vi "LI-U8 - modulus ver2.vi"(3 "Large number - U8 B":T1, 5 "Large number - U8 A":T1) -> (0 "# multiples":T1, 1 "A mod (B)":T1)   [LabVIEW 2012]
doc: "Determines modulus or division remainder of two large numbers (U8 array format).\n\nIterative procedure\na - Is A bigger than B (do subtraction)\n No - output A\n Yes - find the \"base multiplier\" of (A-B) /B . This is done by rounding A-B down so it only keeps highest digit (in base 256) and rounding B up in the same fashion, and dividing the two. Then subtract B * base multiplier from A and go back to top of the loop."
uses:
  User Access Type defs/Large number - U8 array.ctl
panel:
  out "ratio of MSDs":u8
  out "Max # shifts (U8)":u8
  out "Overflow?":bool
  out "A-B":T1
  out "iteration":i32
  # "index 0 = LSD"
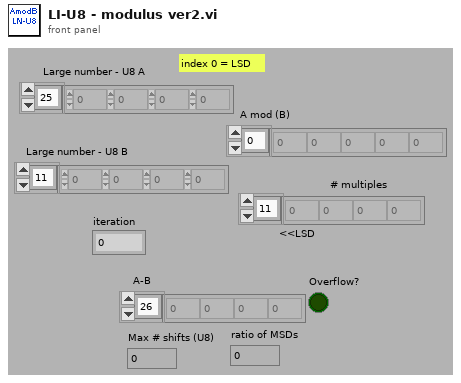
[diagram p1: front panel]
types:
  T1 = typedef "Large number - U8 array.ctl" = u8[]
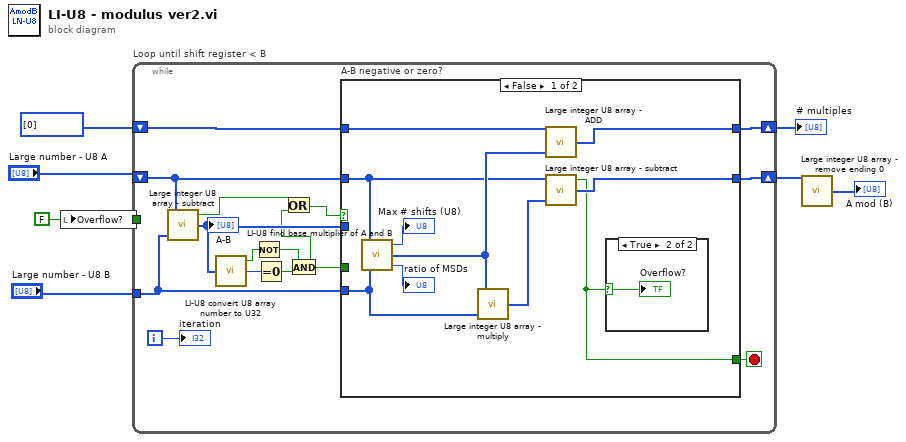
[diagram p0: block diagram]
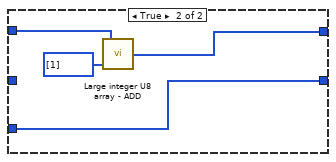
[diagram p4: hidden frame]
diagram:
  w1 = FALSE ("Overflow?")
  n1 = local write "Overflow?"(w1) -> ()
  n2 = while "Loop until shift register < B" {
    shift-right: [w22] -> w5
    shift-left: "Large number - U8 A" -> [w19]
    tunnel: "Large number - U8 B" -> [w21]
    shift-right: [w17] -> w2
    shift-left: T1 [0] ("# multiples") -> [w18]
    tunnel: w1 -> [_]
    i -> [w20]
    stop <- w8 stop-if-true
    n3 = call "Large integer U8 array - subtract.vi"("Large number - U8 B"=w21, "Large number - U8 A"=w19) -> ("A-B"=w16:T1, "Overflow?"=w11:bool)  [unwired: 2 out]
    "A-B" <- w16
    n4 = call "LI-U8 convert U8 array number to U32.vi"("Large number -U8"=w16) -> ("U32"=w15:u32, "Roll-over?"=w14:bool)  [unwired: 3 out]
    n5 = Not(x=w14) -> (.not. x?=w12:bool)
    n6 = Equal To 0?(x=w15) -> (x = 0?=w13:bool)
    n7 = And(x=w12, y=w13) -> (x .and. y?=w10:bool)
    n8 = Or(x=w11, y=w10) -> (x .or. y?=w9:bool)
    n9 = case "A-B negative or zero?" shown="False" w9 {
      selector: w9 -> [_ w34]
      tunnel: [w32 w38] -> w22
      tunnel: w19 -> [w23 w35]
      tunnel: w16 -> [_ w39]
      tunnel: w21 -> [w29 _]
      tunnel: [w30 w36] -> w17
      tunnel: w18 -> [w31 w37]
      tunnel: w10 -> [_ w40]
      tunnel: [w27 w34] -> w8
      frame False {
        n10 = call "LI-U8 find base multiplier of A and B.vi"("Large number - U8 B"=w29, "Large number - U8 A"=w23) -> ("ratio of MSDs"=→"ratio of MSDs":u8, "base multiplier"=w28:T1, "Max # shifts (U8)"=→"Max # shifts (U8)":u8)  [unwired: 1 out]
        n11 = call "Large integer U8 array - multiply.vi"("Large number - U8 2"=w29, "Large number - U8 1"=w28) -> ("Multiplied array"=w26:T1)  [unwired: 3 out]
        n12 = call "Large integer U8 array - ADD.vi"("Large number - U8 2"=w28, "Large number - U8 1"=w31) -> ("Added array"=w30:T1)  [unwired: 3 out]
        n13 = call "Large integer U8 array - subtract.vi"("Large number - U8 B"=w26, "Large number - U8 A"=w23) -> ("A-B"=w32:T1, "Overflow?"=w27:bool)  [unwired: 2 out]
        n14 = case shown="True" w27 {
          selector: w27 -> [_ w33]
          frame False {
          }
          frame True {
            "Overflow?" <- w33
          }
        }
      }
      frame True {
        n15 = case "Remainder zero?" shown="False" w40 {
          tunnel: [w41 w46] -> w38
          tunnel: w39 -> [_ w46]
          tunnel: w37 -> [w42 w45]
          tunnel: [w42 w44] -> w36
          tunnel: w35 -> [w41 _]
          frame False {
          }
          frame True {
            n16 = call "Large integer U8 array - ADD.vi"("Large number - U8 2"=T1 [1], "Large number - U8 1"=w45) -> ("Added array"=w44:T1)  [unwired: 3 out]
          }
        }
      }
    }
    "iteration" <- w20
  }
  "# multiples" <- w2
  n17 = call "Large integer U8 array - remove ending 0.vi"("Large number - U8"=w5) -> ("MSD zeros removed"=→"A mod (B)":T1)  [unwired: 4 out]
